vi "Default Timeout.vi"() -> (0 "Default Timeout":i32=30000)   [LabVIEW 2020, in "serenial.io-ase.test.lvlib"]
uses:
  serenial.io-ase.test.lvlib
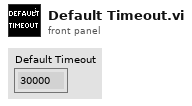
[diagram p1: front panel]
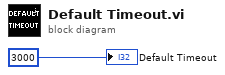
[diagram p0: block diagram]
diagram:
  "Default Timeout" <- 3000
